vi "Move Tail.vi"(6 "Move Delay":u32=25, 7 "XYGraph in":refnum<vi>, 11 "Rope in":cluster{"x":i64, "y":i64}[](array[cluster])) -> (3 "Rope out":cluster{"x":i64, "y":i64}[](array[cluster]), 5 "XY Graph out":refnum<vi>)   [LabVIEW 2021, in "d9.lvlib"]
uses:
  d9.lvlib
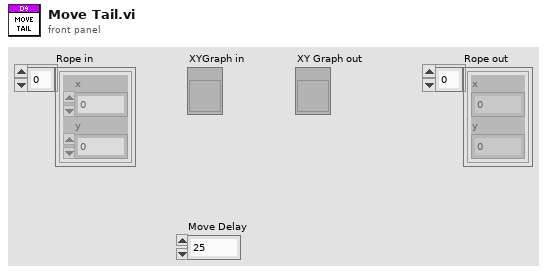
[diagram p1: front panel]
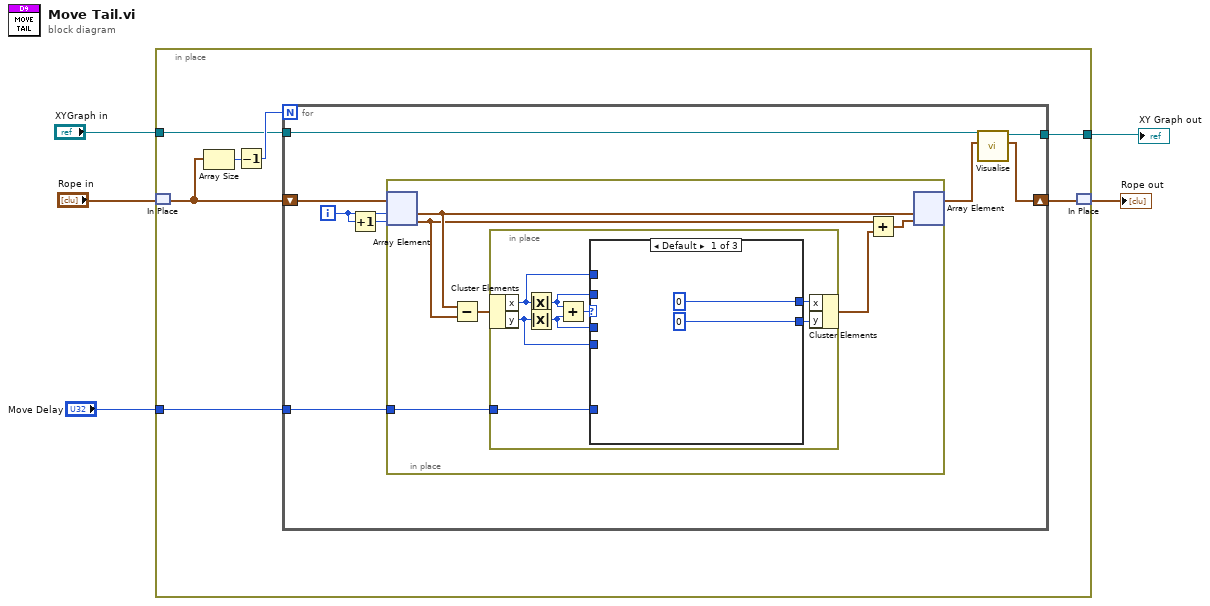
[diagram p0: block diagram]
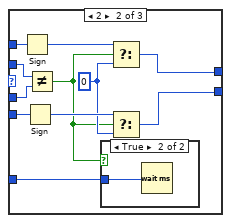
[diagram p2: hidden frame]
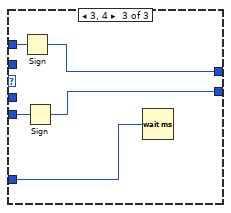
[diagram p4: hidden frame]
diagram:
  n1 = in-place {
    in-place-border: "XYGraph in" -> [w10]
    in-place-border: [w9] -> w4
    in-place-border: "Move Delay" -> [w6]
    n2 = in-place-match #1("Rope in") -> (w8:cluster{"x":i64, "y":i64}[])
    n3 = Array Size(array=w8) -> (size(s)=w12:i32)
    n4 = Decrement(x=w12) -> (x-1=w11:i32)
    n5 = for {
      N: w11 -> [_]
      shift-right: [w14] -> w7
      shift-left: w8 -> [w20]
      tunnel: w10 -> [w17]
      tunnel: [w16] -> w9
      tunnel: w6 -> [w13]
      i -> [w19]
      n6 = Increment(x=w19) -> (x+1=w18:i32)
      n7 = in-place {
        in-place-border: w13 -> [w21]
        n8 = in-place-array #2(w20, w19, w18) -> (w26:cluster{"x":i64, "y":i64}, w25:cluster{"x":i64, "y":i64})
        n9 = Subtract(x=w26, y=w25) -> (x-y=w23:cluster{"x":i64, "y":i64})
        n10 = in-place {
          in-place-border: w21 -> [w27]
          n11 = in-place-cluster #3(w23) -> ("x"=w28:i64, "y"=w29:i64)
          n12 = Absolute Value(x=w28) -> (abs(x)=w30:i64)
          n13 = Absolute Value(x=w29) -> (abs(x)=w31:i64)
          n14 = Add(x=w30, y=w31) -> (x+y=w34:i64)
          n15 = case shown="Default" w34 {
            tunnel: [i64 0 ("y") w41 w50] -> w33
            tunnel: [i64 0 ("x") w42 w51] -> w32
            tunnel: w31 -> [_ w44 _]
            tunnel: w30 -> [_ w45 _]
            tunnel: w29 -> [_ w46 w52]
            tunnel: w28 -> [_ w47 w53]
            tunnel: w27 -> [_ w37 w49]
            frame Default {
            }
            frame 2 {
              w39 = i64 0 ("f")
              n16 = Sign(1:w47) -> (0:w43:i64)
              n17 = Sign(1:w46) -> (0:w40:i64)
              n18 = Not Equal?(x=w45, y=w44) -> (x != y?=w38:bool)
              n19 = case shown="True" w38 {
                tunnel: w37 -> [_ w48]
                frame False {
                }
                frame True {
                  n20 = Wait (ms)(milliseconds to wait=w48) -> ()  [unwired: 1 out]
                }
              }
              n21 = Select(t=w43, s=w38, f=w39) -> (s? t:f=w42:i64)
              n22 = Select(t=w40, s=w38, f=w39) -> (s? t:f=w41:i64)
            }
            frame 3, 4 {
              n23 = Sign(1:w53) -> (0:w51:i64)
              n24 = Sign(1:w52) -> (0:w50:i64)
              n25 = Wait (ms)(milliseconds to wait=w49) -> ()  [unwired: 1 out]
            }
          }
          n26 = in-place-cluster #3("x"=w32, "y"=w33) -> (w22:cluster{"x":i64, "y":i64})
        }
        n27 = Add(x=w25, y=w22) -> (x+y=w24:cluster{"x":i64, "y":i64})
        n28 = in-place-array #2(w26, w24) -> (w15:cluster{"x":i64, "y":i64}[])  [unwired: 2 out]
      }
      n29 = call "Visualise.vi"("Rope in"=w15, "XYGraph in"=w17) -> ("Rope out"=w14:cluster{"x":i64, "y":i64}[], "XY Graph out"=w16:refnum<vi>)  [unwired: 8 in]
    }
    n30 = in-place-match #1(w7) -> (→"Rope out":cluster{"x":i64, "y":i64}[])
  }
  "XY Graph out" <- w4
